vi "LED Lights Subsystem.vi"(8 "error in":errorcluster) -> ()   [LabVIEW 2015]
uses:
  <vilib>/Rock Robotics/SystemInterfaces/i2clib/i2c_bus.ctl
  LED Lights Global.vi
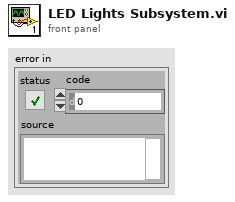
[diagram p1: front panel]
types:
  T1 = typedef "i2c_bus.ctl" = enum16{"I2C On-Board", "I2C MXP", "Invalid"}
  T2 = typedef "LED Lights Ref.ctl" = cluster{"I2CDevRef":T3}
  T3 = typedef "WPI_I2CDevRef.ctl" = cluster{"DevStatus":errorcluster, "Device Address":u8, "Handle":i32, "I2C Bus":T1}
  T4 = typedef "Drive Global Type Def.ctl" = cluster{"Left Drive Motors":T5, "Right Drive Motors":T5}
  T5 = typedef "Master Slave Drive Motors Type Def.ctl" = cluster{"Motor Front":T6, "Motor Back":T6, "Motor Errors":errorcluster, "Motor Top":T6, "Initialized":bool}
  T6 = typedef "Motor Global Type Def.ctl" = cluster{"Motor Error":errorcluster}
  T7 = typedef "NavX Light Global Type Def.ctl" = cluster{"NavX Error":errorcluster, "Initialized":bool}
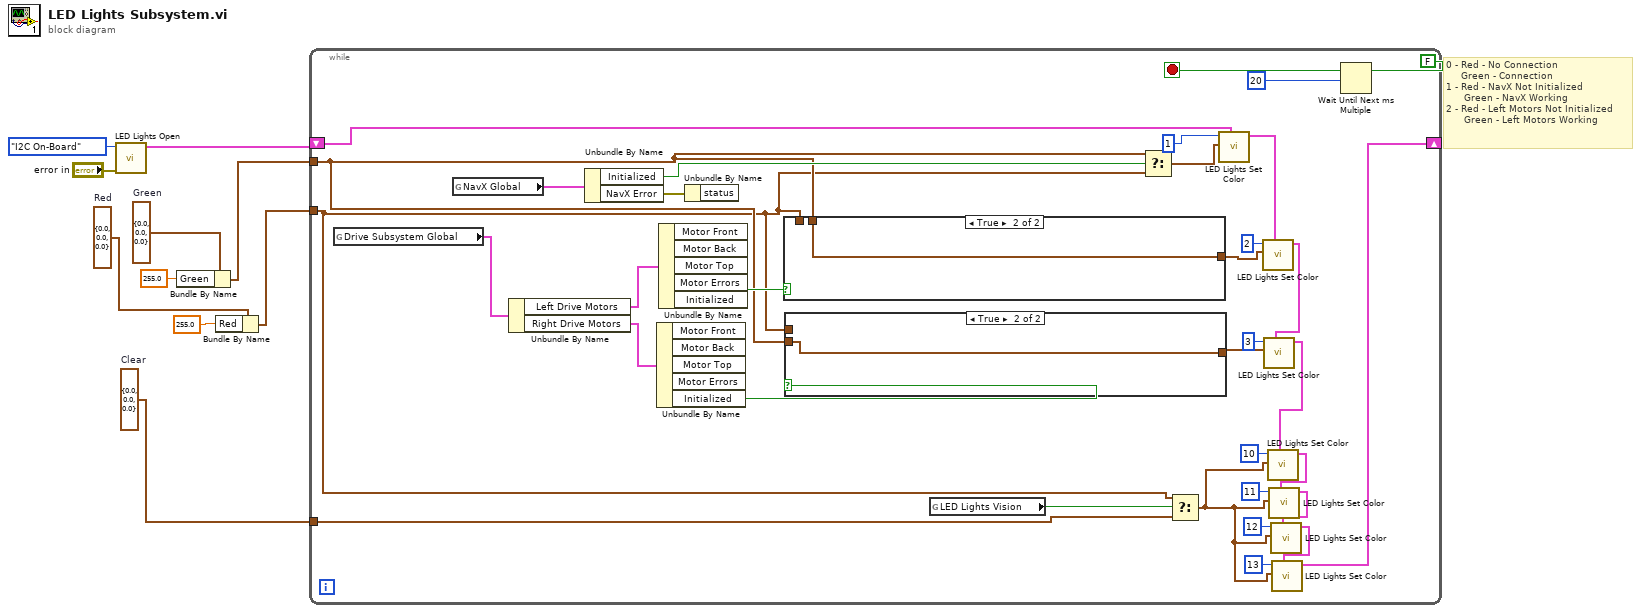
[diagram p0: block diagram]
diagram:
  w1 = cluster{"Red":dbl, "Green":dbl, "Blue":dbl} {"Red"=0.0, "Green"=0.0, "Blue"=0.0}  # Clear
  w4 = cluster{"Red":dbl, "Green":dbl, "Blue":dbl} {"Red"=0.0, "Green"=0.0, "Blue"=0.0}  # Red
  w7 = cluster{"Red":dbl, "Green":dbl, "Blue":dbl} {"Red"=0.0, "Green"=0.0, "Blue"=0.0}  # Green
  # "0 - Red - No Connection\n     Green - Connection\n1 - Red - NavX Not Initialized\n      Green - NavX Working\n2 - Red - Left Motors Not Initialized\n      Green - Left Motors Working"
  n1 = call "LED Lights Open.vi"("error in"="error in", "I2C Bus"=i2c_bus."I2C On-Board") -> ("output cluster"=w8:T2)  [unwired: 8 in, 1 out]
  n2 = Bundle By Name(cluster=w7, "Green"=255.0) -> (w5:cluster{"Red":dbl, "Green":dbl, "Blue":dbl})
  n3 = Bundle By Name(cluster=w4, "Red"=255.0 ("Green")) -> (w2:cluster{"Red":dbl, "Green":dbl, "Blue":dbl})
  n4 = while {
    shift-right: [w12] -> _
    shift-left: w8 -> [w40]
    tunnel: w5 -> [w17]
    tunnel: w2 -> [w11]
    tunnel: w1 -> [w16]
    stop <- FALSE stop-if-true
    n5 = global read "LED Lights Global.vi" "Drive Subsystem Global"() -> (w35:T4)
    n6 = global read "LED Lights Global.vi" "NavX Global"() -> (w38:T7)
    n7 = Unbundle By Name(w35) -> ("Left Drive Motors"=w34:T5, "Right Drive Motors"=w33:T5)
    n8 = Unbundle By Name(w38) -> ("Initialized"=w37:bool, "NavX Error"=w41:errorcluster)
    n9 = Unbundle By Name(w33) -> ("Initialized"=w28:bool)  [unwired: 4 out]
    n10 = Unbundle By Name(w34) -> ("Initialized"=w32:bool)  [unwired: 4 out]
    n11 = Unbundle By Name(w41) -> ()  [unwired: 1 out]
    n12 = case shown="True" w32 {
      tunnel: [w46 w47] -> w29
      tunnel: w11 -> [w46 _]
      tunnel: w17 -> [_ w47]
      frame False {
      }
      frame True {
      }
    }
    n13 = case shown="True" w28 {
      tunnel: [w44 w45] -> w26
      tunnel: w11 -> [w44 _]
      tunnel: w17 -> [_ w45]
      frame False {
      }
      frame True {
      }
    }
    n14 = global read "LED Lights Global.vi" "LED Lights Vision"() -> (w18:bool)
    n15 = Select(t=w17, s=w37, f=w11) -> (s? t:f=w36:cluster{"Red":dbl, "Green":dbl, "Blue":dbl})
    n16 = Select(t=w11, s=w18, f=w16) -> (s? t:f=w19:cluster{"Red":dbl, "Green":dbl, "Blue":dbl})
    n17 = call "LED Lights Set Color.vi"("LED Lights Ref In"=w40, "Color"=w36, "Light ID"=u8 1 ("Light ID 2")) -> ("LED Lights Ref Out"=w31:T2)  [unwired: 7 in, 1 out]
    n18 = call "LED Lights Set Color.vi"("LED Lights Ref In"=w31, "Color"=w29, "Light ID"=u8 2) -> ("LED Lights Ref Out"=w27:T2)  [unwired: 7 in, 1 out]
    n19 = call "LED Lights Set Color.vi"("LED Lights Ref In"=w27, "Color"=w26, "Light ID"=u8 3) -> ("LED Lights Ref Out"=w24:T2)  [unwired: 7 in, 1 out]
    n20 = call "LED Lights Set Color.vi"("LED Lights Ref In"=w24, "Color"=w19, "Light ID"=u8 10) -> ("LED Lights Ref Out"=w15:T2)  [unwired: 7 in, 1 out]
    n21 = call "LED Lights Set Color.vi"("LED Lights Ref In"=w15, "Color"=w19, "Light ID"=u8 11) -> ("LED Lights Ref Out"=w14:T2)  [unwired: 7 in, 1 out]
    n22 = call "LED Lights Set Color.vi"("LED Lights Ref In"=w14, "Color"=w19, "Light ID"=u8 12) -> ("LED Lights Ref Out"=w13:T2)  [unwired: 7 in, 1 out]
    n23 = call "LED Lights Set Color.vi"("LED Lights Ref In"=w13, "Color"=w19, "Light ID"=u8 13) -> ("LED Lights Ref Out"=w12:T2)  [unwired: 7 in, 1 out]
    n24 = Wait Until Next ms Multiple(millisecond multiple=20) -> ()  [unwired: 1 out]
  }
